vi "GOOP_MyComputer_Item_Interface.vi"() -> (3 "InterfaceTable":T1)   [LabVIEW 2014]
uses:
  <resource>/Framework/Providers/API/Item_Interface.ctl
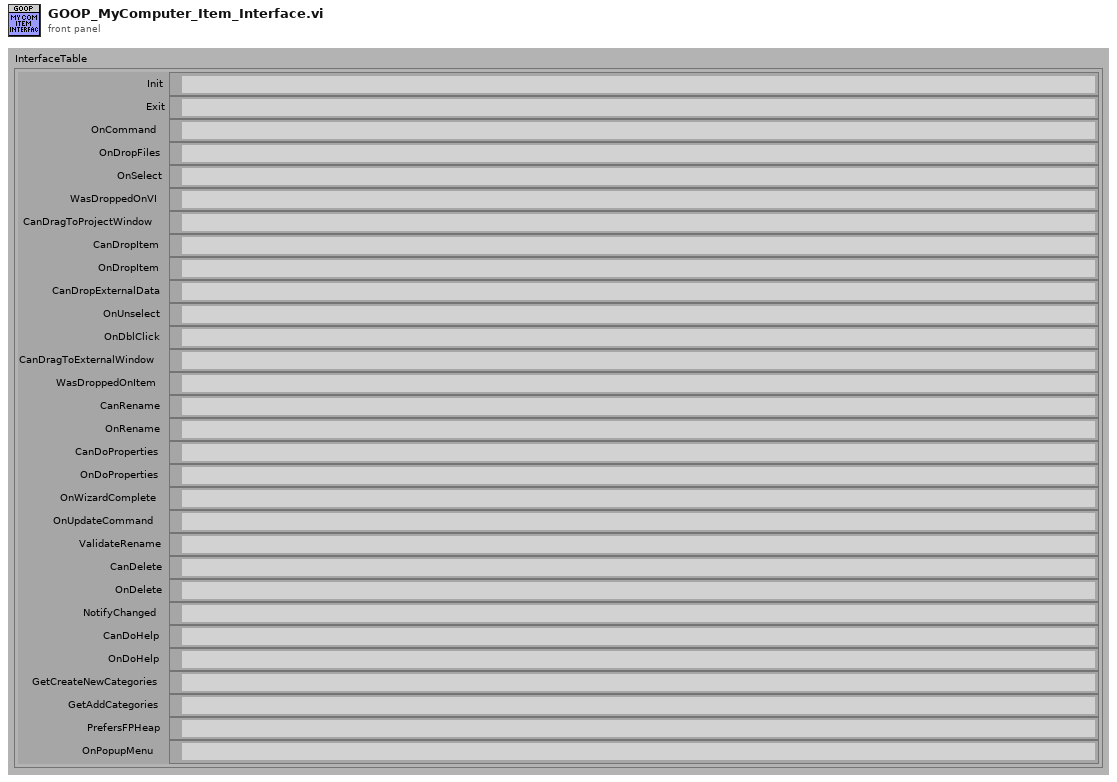
[diagram p1: front panel]
types:
  T1 = typedef "Item_Interface.ctl" = cluster{"Init":path, "Exit":path, "OnCommand":path, "OnDropFiles":path, "OnSelect":path, "WasDroppedOnVI":path, "CanDragToProjectWindow":path, "CanDropItem":path, "OnDropItem":path, "CanDropExternalData":path, "OnUnselect":path, "OnDblClick":path, "CanDragToExternalWindow":path, "WasDroppedOnItem":path, "CanRename":path, "OnRename":path, "CanDoProperties":path, "OnDoProperties":path, "OnWizardComplete":path, "OnUpdateCommand":path, "ValidateRename":path, "CanDelete":path, "OnDelete":path, "NotifyChanged":path, "CanDoHelp":path, "OnDoHelp":path, "GetCreateNewCategories":path, "GetAddCategories":path, "PrefersFPHeap":path, "OnPopupMenu":path}
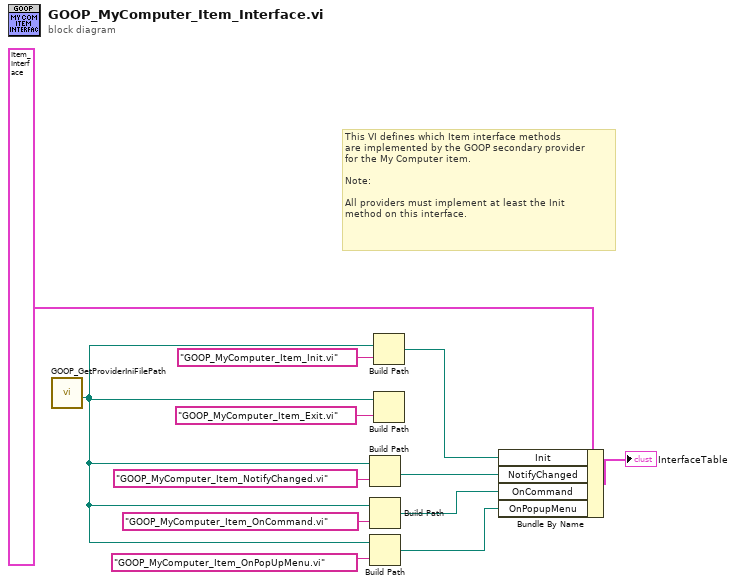
[diagram p0: block diagram]
diagram:
  # "This VI defines which Item interface methods \nare implemented by the GOOP secondary provider \nfor the My Computer item.\n\nNote: \n\nAll providers must implement at least the Init \nmethod on this interface."
  n1 = call <resource>:"GOOP_GetProviderIniFilePath.vi"() -> ("ProviderMainFolder"=w2:path)  [unwired: 10 in, 1 out]
  n2 = Build Path(base path=w2, name or relative path="GOOP_MyComputer_Item_NotifyChanged.vi") -> (appended path=w7:path)
  n3 = Build Path(base path=w2, name or relative path="GOOP_MyComputer_Item_OnCommand.vi") -> (appended path=w5:path)
  n4 = Build Path(base path=w2, name or relative path="GOOP_MyComputer_Item_OnPopUpMenu.vi") -> (appended path=w3:path)
  n5 = Build Path(base path=w2, name or relative path="GOOP_MyComputer_Item_Init.vi") -> (appended path=w10:path)
  n6 = Build Path(base path=w2, name or relative path="GOOP_MyComputer_Item_Exit.vi") -> ()  [unwired: 1 out]
  n7 = Bundle By Name(cluster=T1 {"Init"=path "", "Exit"=path "", "OnCommand"=path "", "OnDropFiles"=path "", "OnSelect"=path "", "WasDroppedOnVI"=path "", "CanDragToProjectWindow"=path "", "CanDropItem"=path "", "OnDropItem"=path "", "CanDropExternalData"=path "", "OnUnselect"=path "", "OnDblClick"=path "", "CanDragToExternalWindow"=path "", "WasDroppedOnItem"=path "", "CanRename"=path "", "OnRename"=path "", "CanDoProperties"=path "", "OnDoProperties"=path "", "OnWizardComplete"=path "", "OnUpdateCommand"=path "", "ValidateRename"=path "", "CanDelete"=path "", "OnDelete"=path "", "NotifyChanged"=path "", "CanDoHelp"=path "", "OnDoHelp"=path "", "GetCreateNewCategories"=path "", "GetAddCategories"=path "", "PrefersFPHeap"=path "", "OnPopupMenu"=path ""} ("InterfaceTable"), "Init"=w10, "NotifyChanged"=w7, "OnCommand"=w5, "OnPopupMenu"=w3) -> (→"InterfaceTable":T1)
